vi "FTW-Test-JSON.vi"() -> ()   [LabVIEW 2015]
uses:
  source/JSON/FTW-JSON.lvclass
panel:
  out "error out":errorcluster
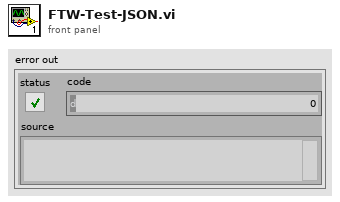
[diagram p1: front panel]
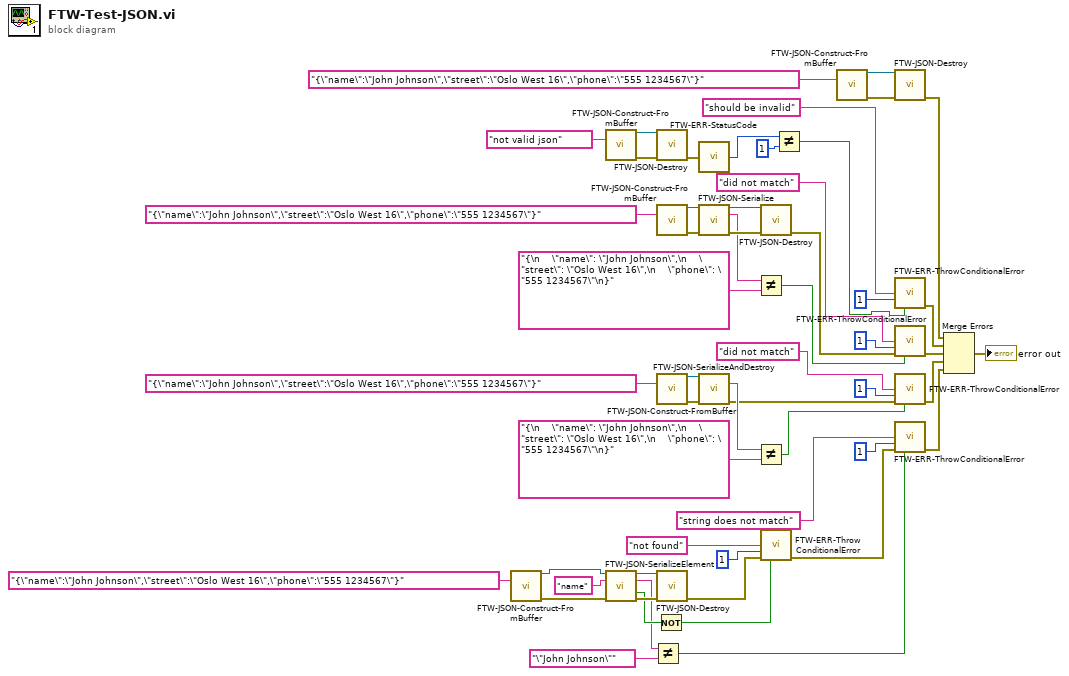
[diagram p0: block diagram]
diagram:
  n1 = call "FTW-JSON-Construct-FromBuffer.vi"("JSON String (UTF-8)"="{\"name\":\"John Johnson\",\"street\":\"Oslo West 16\",\"phone\":\"555 1234567\"}" ("JSON Opject")) -> ("JSON Object"=w36:refnum<class "FTW-JSON.lvclass">, "error out"=w35:errorcluster)  [unwired: 13 in]
  n2 = call "FTW-JSON-Construct-FromBuffer.vi"("JSON String (UTF-8)"="not valid json" ("JSON Opject")) -> ("JSON Object"=w47:refnum<class "FTW-JSON.lvclass">, "error out"=w48:errorcluster)  [unwired: 13 in]
  n3 = call "FTW-JSON-SerializeElement.vi"("JSON Object"=w36, "Key"="name", "error in"=w35) -> ("JSON Object"=w40:refnum<class "FTW-JSON.lvclass">, "Element as JSON String"=w3:string, "Found?"=w9:bool, "error out"=w39:errorcluster)  [unwired: 9 in]
  n4 = Not Equal?(x=w3, y="\"John Johnson\"") -> (x != y?=w2:bool)
  n5 = Not(x=w9) -> (.not. x?=w8:bool)
  n6 = call "FTW-JSON-Destroy.vi"("JSON Object"=w47, "error in"=w48) -> ("error out"=w41:errorcluster)  [unwired: 13 in]
  n7 = call "FTW-JSON-Construct-FromBuffer.vi"("JSON String (UTF-8)"="{\"name\":\"John Johnson\",\"street\":\"Oslo West 16\",\"phone\":\"555 1234567\"}" ("JSON Opject")) -> ("JSON Object"=w53:refnum<class "FTW-JSON.lvclass">, "error out"=w54:errorcluster)  [unwired: 13 in]
  n8 = call "FTW-JSON-Construct-FromBuffer.vi"("JSON String (UTF-8)"="{\"name\":\"John Johnson\",\"street\":\"Oslo West 16\",\"phone\":\"555 1234567\"}" ("JSON Opject")) -> ("JSON Object"=w20:refnum<class "FTW-JSON.lvclass">, "error out"=w19:errorcluster)  [unwired: 13 in]
  n9 = call "FTW-JSON-Destroy.vi"("JSON Object"=w40, "error in"=w39) -> ("error out"=w10:errorcluster)  [unwired: 13 in]
  n10 = call "FTW-ERR-StatusCode.vi"("error to check"=w41) -> ("Code"=w45:i32)
  n11 = call "FTW-JSON-Serialize.vi"("JSON Object"=w53, "error in"=w54) -> ("JSON Object out"=w38:refnum<class "FTW-JSON.lvclass">, "JSON String (UTF-8)"=w28:string, "error out"=w37:errorcluster)  [unwired: 11 in]
  n12 = call "FTW-JSON-SerializeAndDestroy.vi"("JSON Object"=w20, "error in"=w19) -> ("JSON String (UTF-8)"=w22:string, "error out"=w21:errorcluster)  [unwired: 12 in]
  n13 = Not Equal?(x=w28, y="{\n    \"name\": \"John Johnson\",\n    \"street\": \"Oslo West 16\",\n    \"phone\": \"555 1234567\"\n}" ("JSON String (UTF-8)")) -> (x != y?=w25:bool)
  n14 = Not Equal?(x=w22, y="{\n    \"name\": \"John Johnson\",\n    \"street\": \"Oslo West 16\",\n    \"phone\": \"555 1234567\"\n}" ("JSON String (UTF-8)")) -> (x != y?=w24:bool)
  n15 = call "FTW-JSON-Destroy.vi"("JSON Object"=w38, "error in"=w37) -> ("error out"=w33:errorcluster)  [unwired: 13 in]
  n16 = call "FTW-ERR-ThrowConditionalError.vi"("Error Message"="not found", "Error Code"=1, "error in"=w10, "Throw Error?"=w8) -> ("error out"=w4:errorcluster)  [unwired: 11 in]
  n17 = Not Equal?(x=w45, y=1) -> (x != y?=w43:bool)
  n18 = call "FTW-JSON-Construct-FromBuffer.vi"("JSON String (UTF-8)"="{\"name\":\"John Johnson\",\"street\":\"Oslo West 16\",\"phone\":\"555 1234567\"}" ("JSON Opject")) -> ("JSON Object"=w51:refnum<class "FTW-JSON.lvclass">, "error out"=w50:errorcluster)  [unwired: 13 in]
  n19 = call "FTW-JSON-Destroy.vi"("JSON Object"=w51, "error in"=w50) -> ("error out"=w49:errorcluster)  [unwired: 13 in]
  n20 = call "FTW-ERR-ThrowConditionalError.vi"("Error Message"="should be invalid", "Error Code"=1, "Throw Error?"=w43) -> ("error out"=w42:errorcluster)  [unwired: 12 in]
  n21 = call "FTW-ERR-ThrowConditionalError.vi"("Error Message"="did not match", "Error Code"=1, "error in"=w33, "Throw Error?"=w25) -> ("error out"=w26:errorcluster)  [unwired: 11 in]
  n22 = call "FTW-ERR-ThrowConditionalError.vi"("Error Message"="did not match", "Error Code"=1, "error in"=w21, "Throw Error?"=w24) -> ("error out"=w17:errorcluster)  [unwired: 11 in]
  n23 = call "FTW-ERR-ThrowConditionalError.vi"("Error Message"="string does not match", "Error Code"=1, "error in"=w4, "Throw Error?"=w2) -> ("error out"=w5:errorcluster)  [unwired: 11 in]
  n24 = Merge Errors(w49, w42, w26, w17, w5) -> (→"error out":errorcluster)
